vi "Main.vi"() -> ()   [LabVIEW 2014]
doc: "Use this template to build a simple state machine design pattern. Each state executes code and determines which state to transition to."
uses:
  Tipos de onda.ctl
  controls/State.ctl
  controls/Data.ctl
  <vilib>/Waveform/WDTFileIO.llb/ Write Waveform to File.vi
  <vilib>/Analysis/1siggen.llb/Ramp Pattern by Delta.vi
  <vilib>/Waveform/WDTOps.llb/WDT Append Waveforms DBL.vi
  <vilib>/measure/NI_MABase.lvlib
  <vilib>/Waveform/WDTFileIO.llb/Read Waveform from File.vi
  <vilib>/Waveform/WDTFileIO.llb/Export Waveforms To Spreadsheet File (1D).vi
  <vilib>/Analysis/NI_AALBase.lvlib
panel:
  in  "Número de ciclos":dbl
  in  "Tempo de descida":dbl
  in  "Tempo de estabilização":dbl
  in  "Tempo de subida":dbl
  in  "Cortar onda":bool
  in  "Taxa de amostragem":i32
  in  "Amplitude":dbl
  in  "Offset":dbl(slide) scale=0.0..10.0
  out "Ajuste de parâmetros":waveform(dbl)(graph)={"t0"=timestamp(524673.0 s since 1904-01-01), "dt"=0.001, "Y"=[]}
  out "Onda customizada final":waveform(dbl)(graph)
  in  "Duty Cycle (%)":dbl(knob) scale=0.0..100.0
  in  "Fase da onda":dbl(slide) scale=0.0..180.0
  in  "Multiplicador de Frequência":dbl(slide) scale=0.0..1000.0
  in  "Frequência (Hz)":dbl(knob) scale=0.0..10.0
  in  "Tipo de onda":T1
  in  "Gerar nova onda":bool
  in  "Salvar onda":bool
  in  "Histórico de ondas":bool
  in  "Concatenar na onda final":bool
  in  "Sair":bool
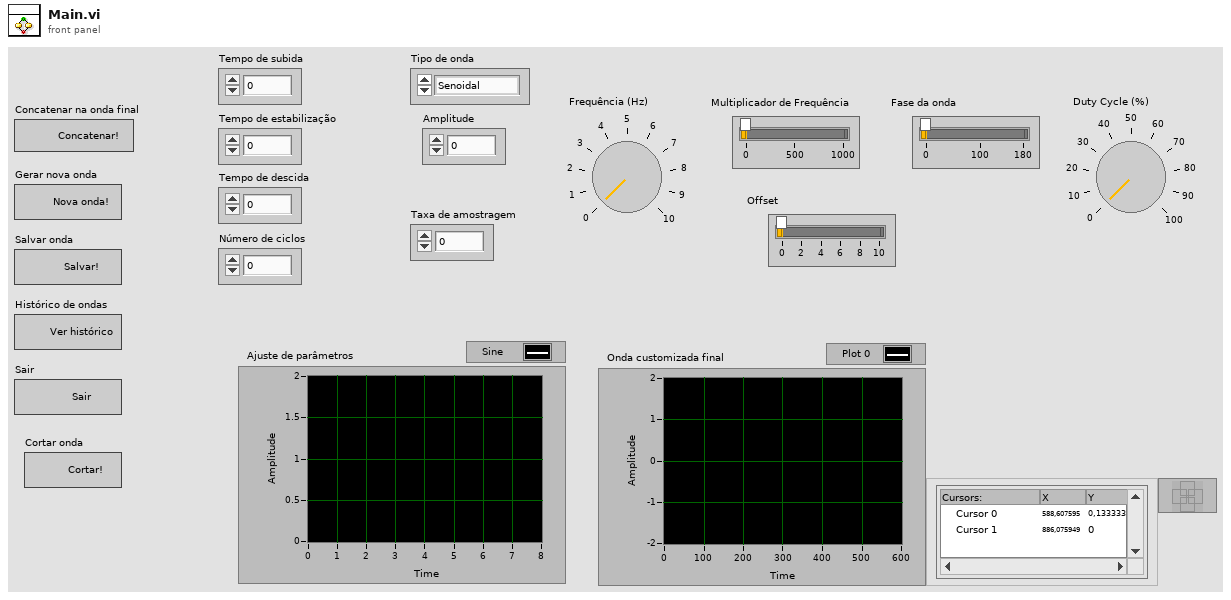
[diagram p1: front panel]
types:
  T1 = typedef "Tipos de onda.ctl" = enum16{"Senoidal", "Quadrada", "Triangular", "Trapezoidal", "Dente de Serra"}
  T2 = typedef "Data.ctl" = cluster{"Boolean <Replace Me>":bool, "String <Replace Me>":string, "Numeric <Replace Me>":dbl, "Onda final":waveform(dbl), "Onda prévia":waveform(dbl), "Tipo de onda":T1, "Frequência (Hz) ":dbl, "Multiplicador de Frequência":dbl, "Fase da onda":dbl, "Duty Cycle (%)":dbl, "Offset":dbl, "Amplitude":dbl, "Taxa de amostragem":i32, "Remove Button":bool, "Tempo de subida":dbl, "Tempo de estabilização":dbl, "Tempo de descida":dbl, "Número de ciclos":dbl}
  T3 = typedef "State.ctl" = enum16{"Inicializar", "Aguardar evento", "Concatenar na onda final", "Ajustar onda prévia", "Cortar onda", "Gerar nova onda", "Salvar onda", "Histórico de ondas", "Sair"}
  T4 = typedef "LVCursorListTypeDef.ctl" = cluster{"Name":string, "Color":u32, "Style":u8, "Point Style":u8, "Name Visible":bool, "Allow Drag":bool, "Cursor Mode":u32, "Plot":i32, "Index":i32, "Position":cluster{"X":dbl, "Y":dbl}, "X Scale":u32, "Y Scale":u32, "Watch Plots":i32[], "Watch All Plots":bool, "Plot Area":i32, "Label Offset":cluster{"X":dbl, "Y":dbl}}[]
  T5 = cluster{"CrsrList[0]":cluster{"Name":string, "Color":u32, "Style":u8, "Point Style":u8, "Name Visible":bool, "Allow Drag":bool, "Cursor Mode":u32, "Plot":i32, "Index":i32, "Position":cluster{"X":dbl, "Y":dbl}, "X Scale":u32, "Y Scale":u32, "Watch Plots":i32[], "Watch All Plots":bool, "Plot Area":i32, "Label Offset":cluster{"X":dbl, "Y":dbl}}, "CrsrList[1]":cluster{"Name":string, "Color":u32, "Style":u8, "Point Style":u8, "Name Visible":bool, "Allow Drag":bool, "Cursor Mode":u32, "Plot":i32, "Index":i32, "Position":cluster{"X":dbl, "Y":dbl}, "X Scale":u32, "Y Scale":u32, "Watch Plots":i32[], "Watch All Plots":bool, "Plot Area":i32, "Label Offset":cluster{"X":dbl, "Y":dbl}}, "CrsrList[2]":cluster{"Name":string, "Color":u32, "Style":u8, "Point Style":u8, "Name Visible":bool, "Allow Drag":bool, "Cursor Mode":u32, "Plot":i32, "Index":i32, "Position":cluster{"X":dbl, "Y":dbl}, "X Scale":u32, "Y Scale":u32, "Watch Plots":i32[], "Watch All Plots":bool, "Plot Area":i32, "Label Offset":cluster{"X":dbl, "Y":dbl}}, "CrsrList[3]":cluster{"Name":string, "Color":u32, "Style":u8, "Point Style":u8, "Name Visible":bool, "Allow Drag":bool, "Cursor Mode":u32, "Plot":i32, "Index":i32, "Position":cluster{"X":dbl, "Y":dbl}, "X Scale":u32, "Y Scale":u32, "Watch Plots":i32[], "Watch All Plots":bool, "Plot Area":i32, "Label Offset":cluster{"X":dbl, "Y":dbl}}, "CrsrList[4]":cluster{"Name":string, "Color":u32, "Style":u8, "Point Style":u8, "Name Visible":bool, "Allow Drag":bool, "Cursor Mode":u32, "Plot":i32, "Index":i32, "Position":cluster{"X":dbl, "Y":dbl}, "X Scale":u32, "Y Scale":u32, "Watch Plots":i32[], "Watch All Plots":bool, "Plot Area":i32, "Label Offset":cluster{"X":dbl, "Y":dbl}}, "CrsrList[5]":cluster{"Name":string, "Color":u32, "Style":u8, "Point Style":u8, "Name Visible":bool, "Allow Drag":bool, "Cursor Mode":u32, "Plot":i32, "Index":i32, "Position":cluster{"X":dbl, "Y":dbl}, "X Scale":u32, "Y Scale":u32, "Watch Plots":i32[], "Watch All Plots":bool, "Plot Area":i32, "Label Offset":cluster{"X":dbl, "Y":dbl}}, "CrsrList[6]":cluster{"Name":string, "Color":u32, "Style":u8, "Point Style":u8, "Name Visible":bool, "Allow Drag":bool, "Cursor Mode":u32, "Plot":i32, "Index":i32, "Position":cluster{"X":dbl, "Y":dbl}, "X Scale":u32, "Y Scale":u32, "Watch Plots":i32[], "Watch All Plots":bool, "Plot Area":i32, "Label Offset":cluster{"X":dbl, "Y":dbl}}, "CrsrList[7]":cluster{"Name":string, "Color":u32, "Style":u8, "Point Style":u8, "Name Visible":bool, "Allow Drag":bool, "Cursor Mode":u32, "Plot":i32, "Index":i32, "Position":cluster{"X":dbl, "Y":dbl}, "X Scale":u32, "Y Scale":u32, "Watch Plots":i32[], "Watch All Plots":bool, "Plot Area":i32, "Label Offset":cluster{"X":dbl, "Y":dbl}}, "CrsrList[8]":cluster{"Name":string, "Color":u32, "Style":u8, "Point Style":u8, "Name Visible":bool, "Allow Drag":bool, "Cursor Mode":u32, "Plot":i32, "Index":i32, "Position":cluster{"X":dbl, "Y":dbl}, "X Scale":u32, "Y Scale":u32, "Watch Plots":i32[], "Watch All Plots":bool, "Plot Area":i32, "Label Offset":cluster{"X":dbl, "Y":dbl}}}
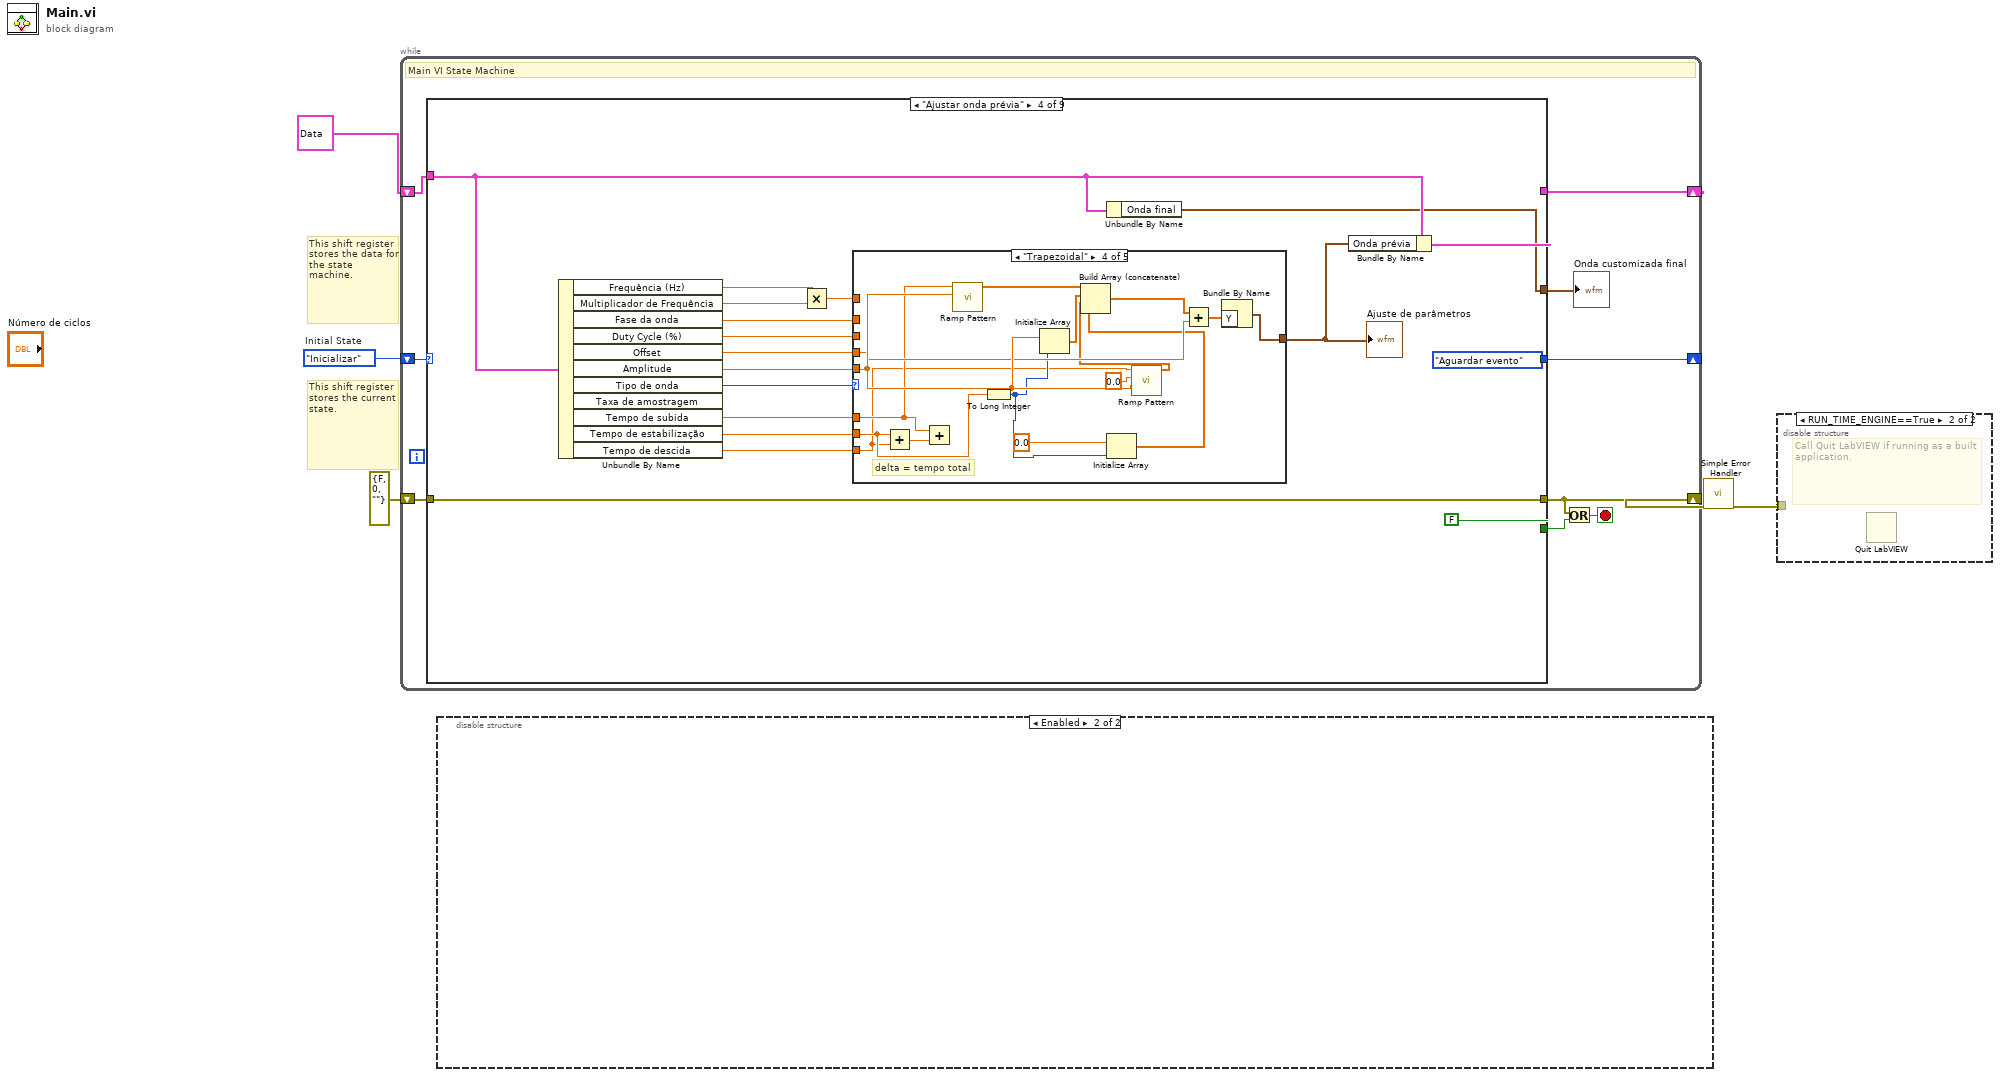
[diagram p0: block diagram]
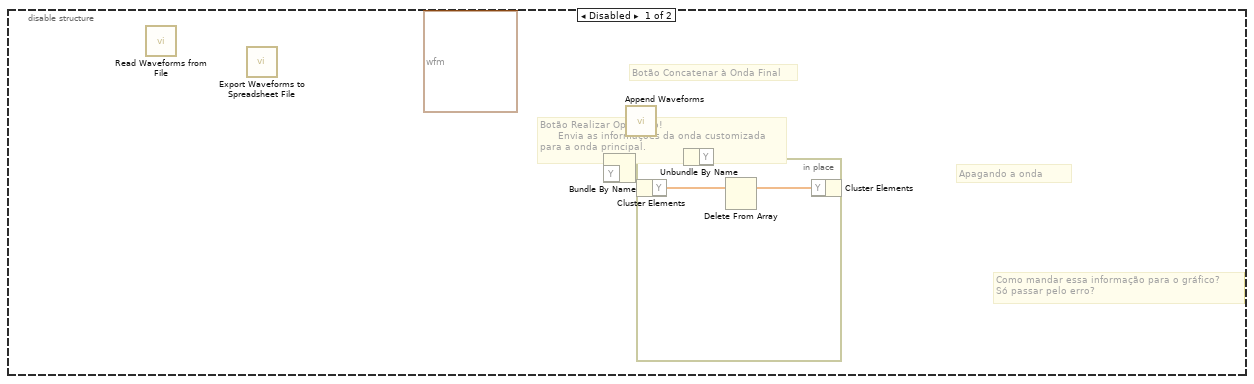
[diagram p2: hidden frame]
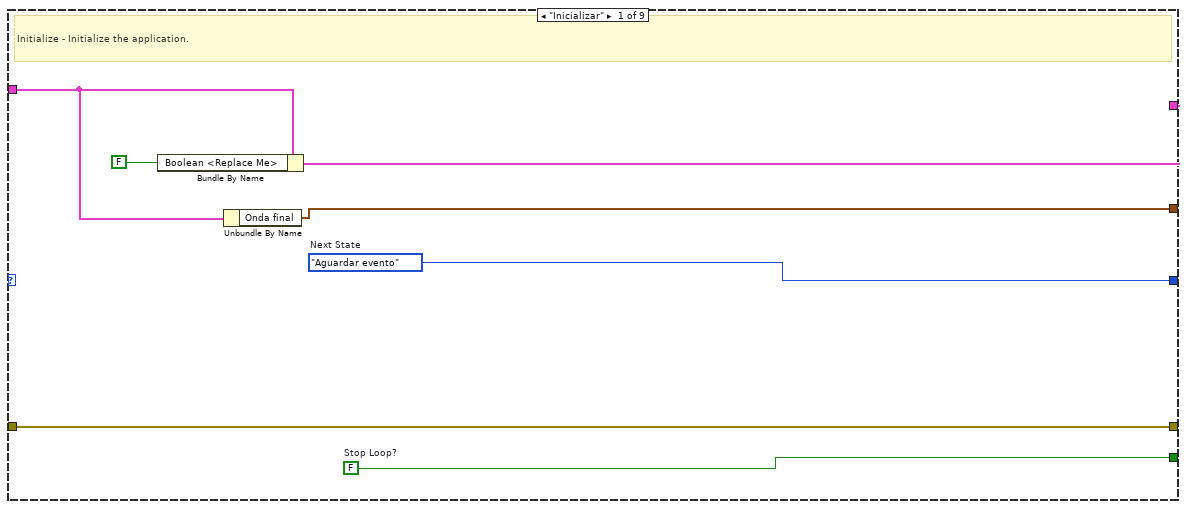
[diagram p4: hidden frame]
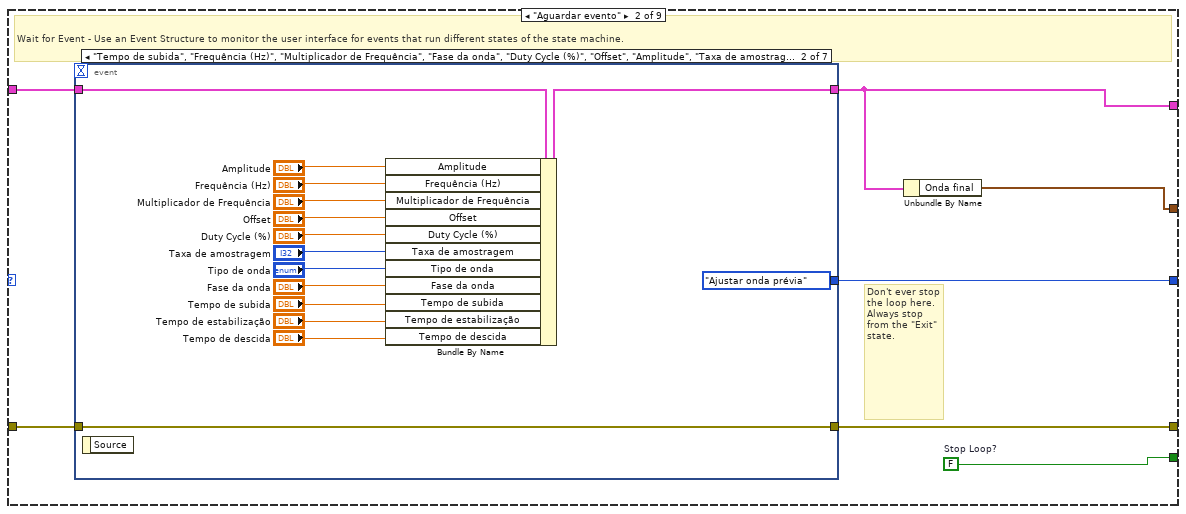
[diagram p5: hidden frame]
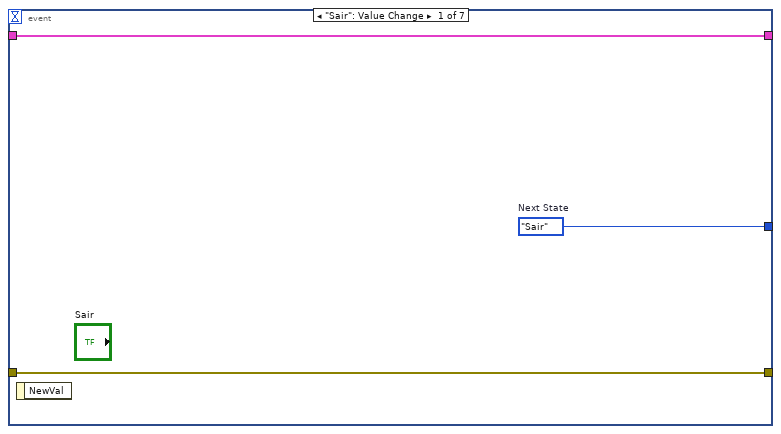
[diagram p6: hidden frame]
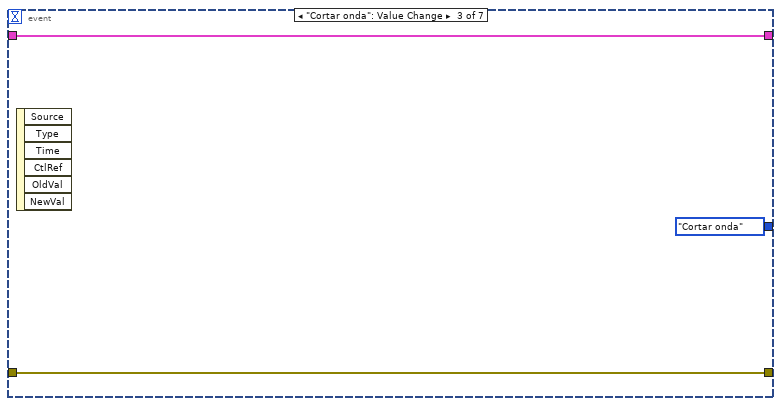
[diagram p7: hidden frame]
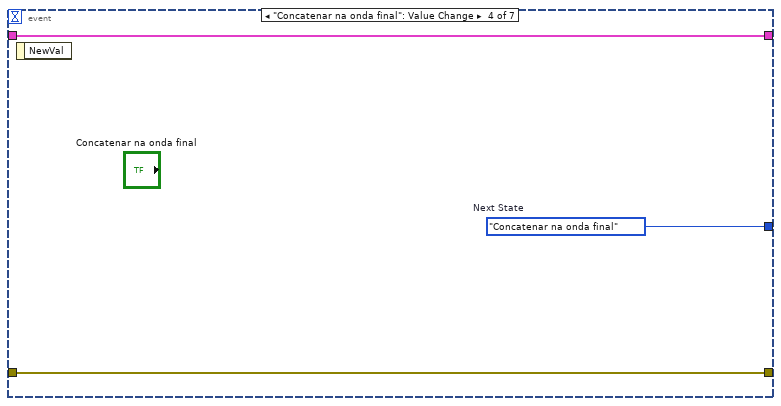
[diagram p8: hidden frame]
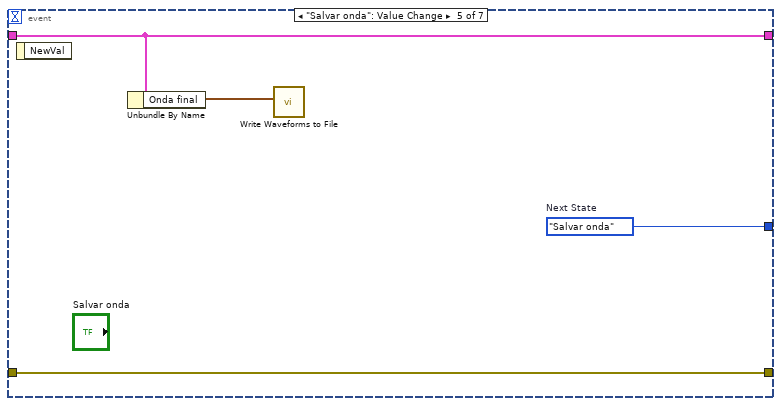
[diagram p9: hidden frame]
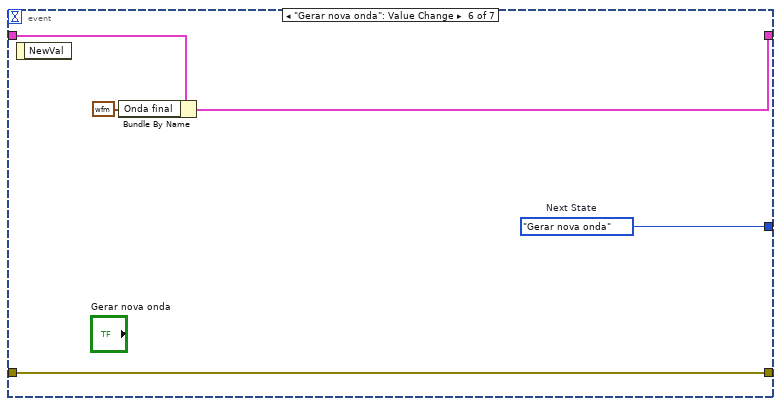
[diagram p10: hidden frame]
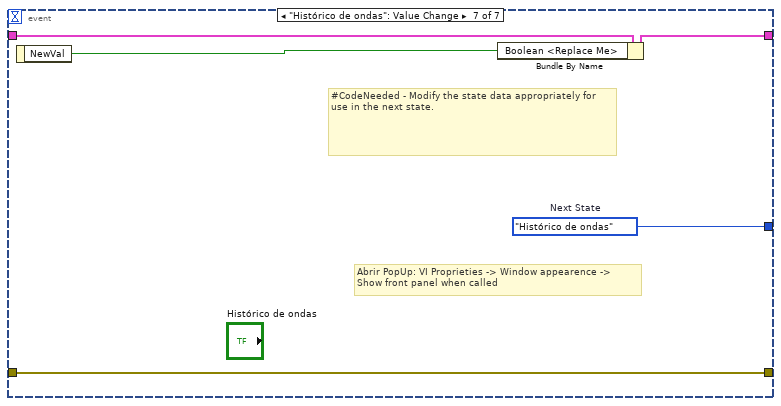
[diagram p11: hidden frame]
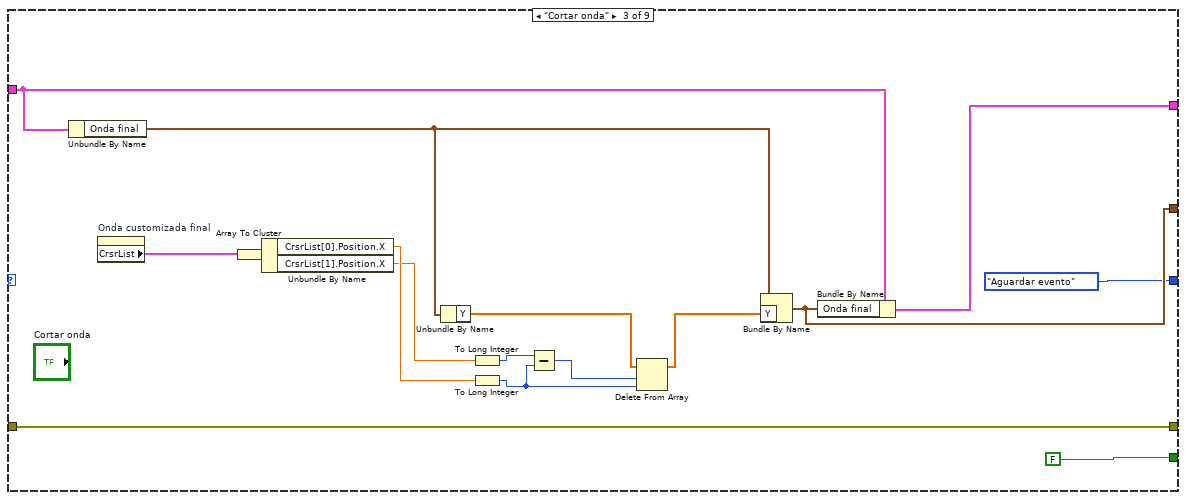
[diagram p12: hidden frame]
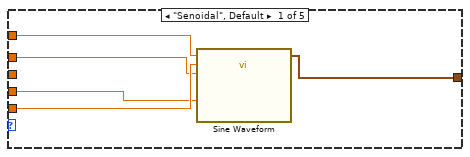
[diagram p13: hidden frame]
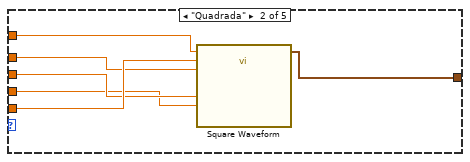
[diagram p14: hidden frame]
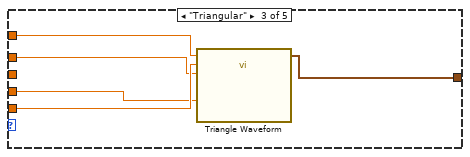
[diagram p15: hidden frame]
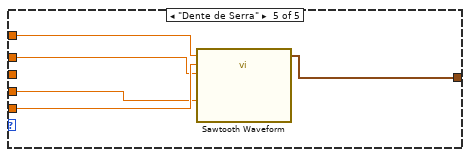
[diagram p16: hidden frame]
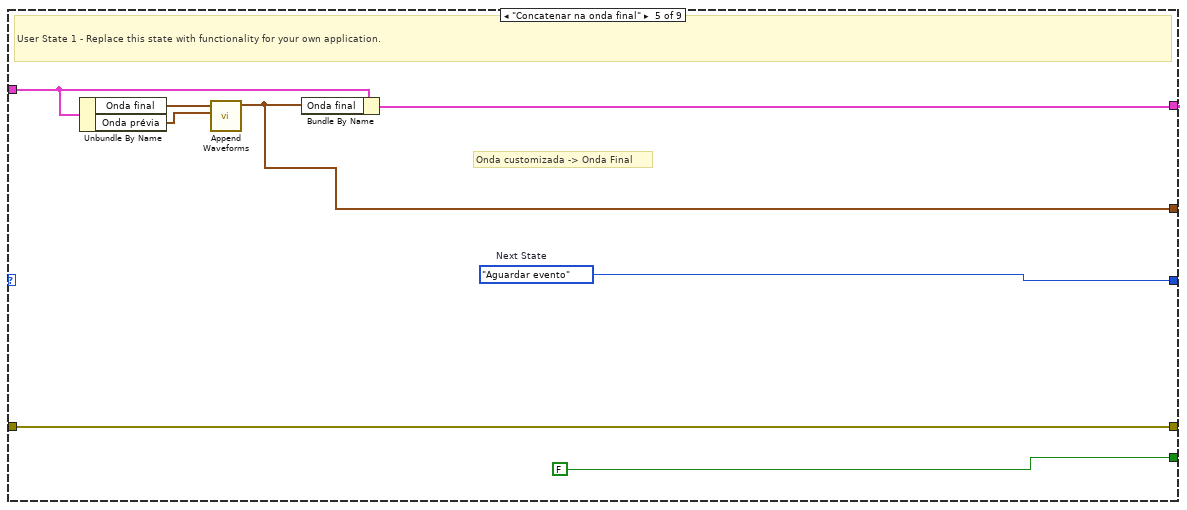
[diagram p17: hidden frame]
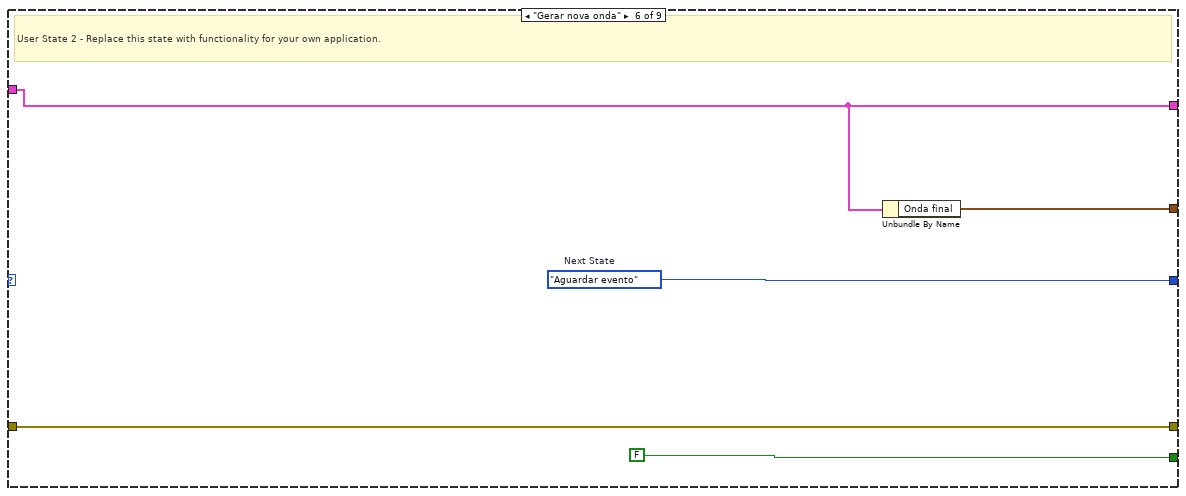
[diagram p18: hidden frame]
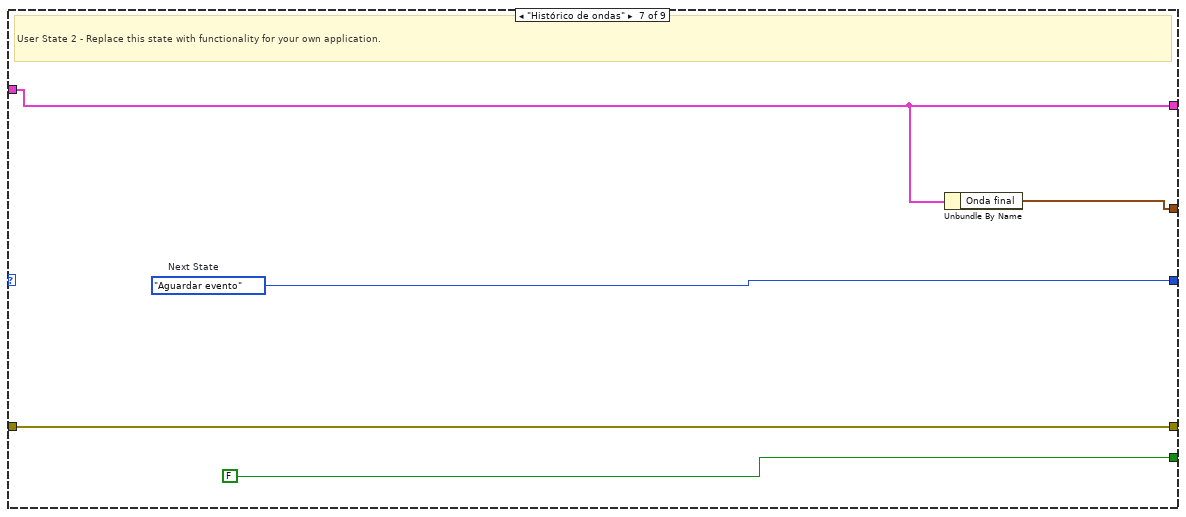
[diagram p19: hidden frame]
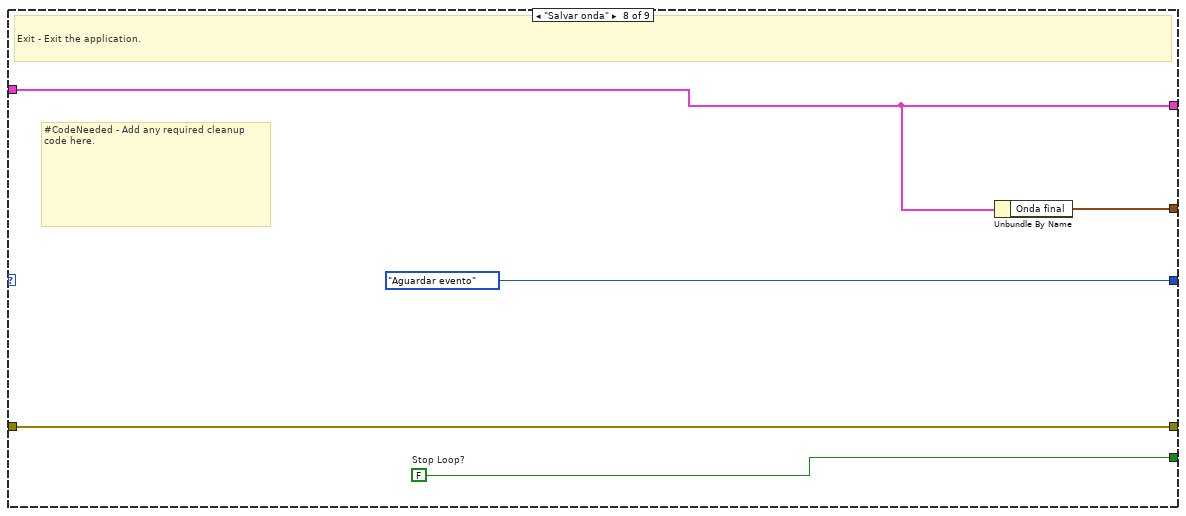
[diagram p20: hidden frame]
diagram:
  w5 = State."Inicializar"  # Initial State
  # "This shift register stores the data for the state machine."
  # "This shift register stores the current state."
  n1 = while {
    shift-right: [w13] -> _
    shift-left: w5 -> [w14]
    shift-right: [w11] -> _
    shift-left: T2 {"Boolean <Replace Me>"=FALSE, "String <Replace Me>"="", "Numeric <Replace Me>"=0.0, "Onda final"={"t0"=timestamp(0 s since 1904-01-01), "dt"=1.0, "Y"=[]}, "Onda prévia"={"t0"=timestamp(0 s since 1904-01-01), "dt"=1.0, "Y"=[]}, "Tipo de onda"=enum."Senoidal", "Frequência (Hz) "=0.0, "Multiplicador de Frequência"=0.0, "Fase da onda"=0.0, "Duty Cycle (%)"=0.0, "Offset"=0.0, "Amplitude"=0.0, "Taxa de amostragem"=0, "Remove Button"=FALSE, "Tempo de subida"=0.0, "Tempo de estabilização"=0.0, "Tempo de descida"=0.0, "Número de ciclos"=0.0} ("Data") -> [w12]
    shift-right: [w8] -> w2
    shift-left: errorcluster {"status"=FALSE, "code"=0, "source"=""} ("error constant") -> [w10]
    stop <- w9 stop-if-true
    # "Main VI State Machine"
    n2 = case shown="\"Ajustar onda prévia\"" w14 {
      tunnel: [w21 w28 State."Aguardar evento" ("(Value Not Used)") State."Aguardar evento" ("(Value Not Used)") w145 w150 w155 State."Aguardar evento" w165] -> w13
      tunnel: [w20 w27 FALSE ("Stop Loop?") FALSE FALSE ("Stop Loop?") FALSE ("Stop Loop?") FALSE ("Stop Loop?") w159 w164] -> w7
      tunnel: w12 -> [w16 w26 w71 w90 w139 w146 w151 w156 w161]
      tunnel: [w19 w23 w70 w94 w142 w146 w151 w156 w161] -> w11
      tunnel: w10 -> [w17 w24 w79 w100 w143 w148 w153 w158 w163]
      tunnel: [w17 w25 w79 w100 w143 w148 w153 w158 w163] -> w8
      tunnel: [w15 w22 w69 w89 w138 w147 w152 w157 w162] -> w6
      frame "Inicializar" {
        w20 = FALSE  # Stop Loop?
        w21 = State."Aguardar evento"  # Next State
        # "Initialize - Initialize the application."
        n3 = Bundle By Name(cluster=w16, "Boolean <Replace Me>"=FALSE ("Replace_Me_Boolean")) -> (w19:T2)
        n4 = Unbundle By Name(w16) -> ("Onda final"=w15:waveform(dbl))
      }
      frame "Aguardar evento" {
        w27 = FALSE  # Stop Loop?
        # "Don't ever stop the loop here. Always stop from the \"Exit\" state."
        # "Wait for Event - Use an Event Structure to monitor the user interface for events that run different states of the state machine."
        n5 = event shown="[1] \"Tempo de subida\", \"Frequência (Hz)\", \"Multiplicador de Frequência\", \"Fase da onda\", \"Duty Cycle (%)\", \"Offset\", \"Amplitude\", \"Taxa de amostragem\", \"Tempo de estabilização\", \"Tempo de descida\": Value Change" {
          selector: _ -> [_ _ _ _ _ _ _]
          dyn-events: _ -> [_ _ _ _ _ _ _]
          timeout: _ -> [_ _ _ _ _ _ _]
          tunnel: [w31 State."Ajustar onda prévia" ("Next State") State."Cortar onda" ("Next State") w52 w56 w61 w66] -> w28
          tunnel: w26 -> [w30 w46 w49 w50 w53 w59 w65]
          tunnel: [w30 w43 w49 w50 w53 w57 w64] -> w23
          tunnel: w24 -> [w29 w45 w48 w51 w55 w60 w63]
          tunnel: [w29 w45 w48 w51 w55 w60 w63] -> w25
          event "Sair": Value Change {
            w31 = State."Sair"  # Next State
            n6 = event-data() -> ()  [unwired: 1 in, 1 out]
          }
          event "Tempo de subida", "Frequência (Hz)", "Multiplicador de Frequência", "Fase da onda", "Duty Cycle (%)", "Offset", "Amplitude", "Taxa de amostragem", "Tempo de estabilização", "Tempo de descida": Value Change {
            n7 = event-data() -> ()  [unwired: 1 in, 1 out]
            n8 = Bundle By Name(cluster=w46, "Amplitude"="Amplitude", "Frequência (Hz)"="Frequência (Hz)", "Multiplicador de Frequência"="Multiplicador de Frequência", "Offset"="Offset", "Duty Cycle (%)"="Duty Cycle (%)", "Taxa de amostragem"="Taxa de amostragem", "Tipo de onda"="Tipo de onda", "Fase da onda"="Fase da onda", "Tempo de subida"="Tempo de subida", "Tempo de estabilização"="Tempo de estabilização", "Tempo de descida"="Tempo de descida") -> (w43:T2)
          }
          event "Cortar onda": Value Change {
            n9 = event-data() -> ()  [unwired: 1 in, 6 out]
          }
          event "Concatenar na onda final": Value Change {
            w52 = State."Concatenar na onda final"  # Next State
            n10 = event-data() -> ()  [unwired: 1 in, 1 out]
          }
          event "Salvar onda": Value Change {
            w56 = State."Salvar onda"  # Next State
            n11 = event-data() -> ()  [unwired: 1 in, 1 out]
            n12 = Unbundle By Name(w53) -> ("Onda final"=w54:waveform(dbl))
            n13 = call-poly <vilib>:"Write Waveforms to File.vi"("waveform"=w54) -> ()  [unwired: 9 in, 2 out]
          }
          event "Gerar nova onda": Value Change {
            w61 = State."Gerar nova onda"  # Next State
            n14 = event-data() -> ()  [unwired: 1 in, 1 out]
            n15 = Bundle By Name(cluster=w59, "Onda final"=waveform(dbl) {"t0"=timestamp(0 s since 1904-01-01), "dt"=1.0, "Y"=[]}) -> (w57:T2)
          }
          event "Histórico de ondas": Value Change {
            w66 = State."Histórico de ondas"  # Next State
            # "Abrir PopUp: VI Proprieties -> Window appearence ->\nShow front panel when called"
            # "#CodeNeeded - Modify the state data appropriately for use in the next state."
            n16 = event-data() -> ("NewVal"=w62:bool)  [unwired: 1 in]
            n17 = Bundle By Name(cluster=w65, "Boolean <Replace Me>"=w62) -> (w64:T2)
          }
        }
        n18 = Unbundle By Name(w23) -> ("Onda final"=w22:waveform(dbl))
      }
      frame "Cortar onda" {
        n19 = Unbundle By Name(w71) -> ("Onda final"=w72:waveform(dbl))
        n20 = property on="Onda customizada final" class="WFGraph (strict)"() -> ("CrsrList"=w81:T4)  [unwired: 2 in, 2 out]
        n21 = Array To Cluster(array=w81) -> (cluster=w80:T5)
        n22 = Unbundle By Name(w80) -> ("CrsrList[0].Position.X"=w78:dbl, "CrsrList[1].Position.X"=w77:dbl)
        n23 = Unbundle By Name(w72) -> ("Y"=w82:dbl[])
        n24 = To Long Integer(number=w77) -> (32bit integer=w76:i32)
        n25 = To Long Integer(number=w78) -> (32bit integer=w75:i32)
        n26 = Subtract(x=w76, y=w75) -> (x-y=w74:i32)
        n27 = Delete From Array(array=w82, length=w74, index=w75) -> (array with subset deleted=w73:dbl[])  [unwired: 1 out]
        n28 = Bundle By Name(cluster=w72, "Y"=w73) -> (w69:waveform(dbl))
        n29 = Bundle By Name(cluster=w71, "Onda final"=w69) -> (w70:T2)
      }
      frame "Ajustar onda prévia" {
        n30 = Unbundle By Name(w90) -> ("Frequência (Hz)"=w88:dbl, "Multiplicador de Frequência"=w87:dbl, "Fase da onda"=w93:dbl, "Duty Cycle (%)"=w92:dbl, "Offset"=w91:dbl, "Amplitude"=w98:dbl, "Tipo de onda"=w99:T1, "Tempo de subida"=w85:dbl, "Tempo de estabilização"=w84:dbl, "Tempo de descida"=w83:dbl)  [unwired: 1 out]
        n31 = Multiply(x=w88, y=w87) -> (x*y=w86:dbl)
        n32 = case shown="\"Trapezoidal\"" w99 {
          tunnel: [w105 w111 w116 w127 w137] -> w95
          tunnel: w98 -> [w104 w110 w115 w130 w136]
          tunnel: w86 -> [w103 w109 w114 _ w135]
          tunnel: w93 -> [w102 w108 w113 _ w134]
          tunnel: w92 -> [_ w107 _ _ _]
          tunnel: w91 -> [w101 w106 w112 w128 w133]
          tunnel: w85 -> [_ _ _ w118 _]
          tunnel: w84 -> [_ _ _ w131 _]
          tunnel: w83 -> [_ _ _ w117 _]
          frame "Senoidal", Default {
            n33 = call <vilib>:"Sine Waveform.vi"("offset"=w101, "phase"=w102, "amplitude"=w104, "frequency"=w103) -> ("signal out"=w105:waveform(dbl))  [unwired: 6 in, 1 out]
          }
          frame "Quadrada" {
            n34 = call <vilib>:"Square Waveform.vi"("duty cycle (%)"=w107, "offset"=w106, "phase"=w108, "amplitude"=w110, "frequency"=w109) -> ("signal out"=w111:waveform(dbl))  [unwired: 5 in, 1 out]
          }
          frame "Triangular" {
            n35 = call <vilib>:"Triangle Waveform.vi"("offset"=w112, "phase"=w113, "amplitude"=w115, "frequency"=w114) -> ("signal out"=w116:waveform(dbl))  [unwired: 6 in, 1 out]
          }
          frame "Trapezoidal" {
            # "delta = tempo total"
            n36 = Add(x=w131, y=w117) -> (x+y=w132:dbl)
            n37 = Add(x=w118, y=w132) -> ()  [unwired: 1 out]
            n38 = call-poly <vilib>:"Ramp Pattern.vi"("end"=w130, "delta"=w118) -> ("Ramp Pattern"=w126:dbl[])  [unwired: 7 in, 2 out]
            n39 = To Long Integer(number=w131) -> (32bit integer=w120:i32)
            n40 = Initialize Array(w130, w120) -> (w125:dbl[])
            n41 = Initialize Array(0.0 ("element"), w120) -> (w119:dbl[])
            n42 = call-poly <vilib>:"Ramp Pattern.vi"("start"=w130, "end"=0.0, "delta"=w117) -> ("Ramp Pattern"=w124:dbl[])  [unwired: 6 in, 2 out]
            n43 = Build Array (concatenate)(w126, w125, w124, w119) -> (w123:dbl[])
            n44 = Add(x=w123, y=w128) -> (x+y=w122:dbl[])
            n45 = Bundle By Name("Y"=w122) -> (w127:waveform(dbl))  [unwired: 1 in]
          }
          frame "Dente de Serra" {
            n46 = call <vilib>:"Sawtooth Waveform.vi"("offset"=w133, "phase"=w134, "amplitude"=w136, "frequency"=w135) -> ("signal out"=w137:waveform(dbl))  [unwired: 6 in, 1 out]
          }
        }
        "Ajuste de parâmetros" <- w95
        n47 = Unbundle By Name(w90) -> ("Onda final"=w89:waveform(dbl))
        n48 = Bundle By Name(cluster=w90, "Onda prévia"=w95) -> (w94:T2)
      }
      frame "Concatenar na onda final" {
        w145 = State."Aguardar evento"  # Next State
        # "Onda customizada -> Onda Final"
        # "User State 1 - Replace this state with functionality for your own application."
        n49 = Unbundle By Name(w139) -> ("Onda final"=w141:waveform(dbl), "Onda prévia"=w140:waveform(dbl))
        n50 = call-poly <vilib>:"Append Waveforms.vi"("waveform B"=w140, "waveform A"=w141) -> ("waveform out"=w138:waveform(dbl))  [unwired: 8 in, 1 out]
        n51 = Bundle By Name(cluster=w139, "Onda final"=w138) -> (w142:T2)
      }
      frame "Gerar nova onda" {
        w150 = State."Aguardar evento"  # Next State
        # "User State 2 - Replace this state with functionality for your own application."
        n52 = Unbundle By Name(w146) -> ("Onda final"=w147:waveform(dbl))
      }
      frame "Histórico de ondas" {
        w155 = State."Aguardar evento"  # Next State
        # "User State 2 - Replace this state with functionality for your own application."
        n53 = Unbundle By Name(w151) -> ("Onda final"=w152:waveform(dbl))
      }
      frame "Salvar onda" {
        w159 = FALSE  # Stop Loop?
        # "#CodeNeeded - Add any required cleanup code here."
        # "Exit - Exit the application."
        n54 = Unbundle By Name(w156) -> ("Onda final"=w157:waveform(dbl))
      }
      frame "Sair" {
        w164 = TRUE  # Stop Loop?
        w165 = State."Sair"  # (Value Not Used)
        # "Exit - Exit the application."
        n55 = Unbundle By Name(w161) -> ("Onda final"=w162:waveform(dbl))
      }
    }
    "Onda customizada final" <- w6
    n56 = Or(x=w8, y=w7) -> (x .or. y?=w9:bool)
  }
  n57 = disable-structure shown="Enabled" {
    frame Disabled {
      (unwired) waveform(dbl) {"t0"=timestamp(0 s since 1904-01-01), "dt"=1.0, "Y"=[]} ("Waveform")
      # "Botão Concatenar à Onda Final"
      # "Como mandar essa informação para o gráfico?\nSó passar pelo erro?"
      # "Apagando a onda"
      # "Botão Realizar Operação!\n      Envia as informações da onda customizada\npara a onda principal."
      n58 = call-poly <vilib>:"Read Waveforms from File.vi"() -> ()  [unwired: 6 in, 4 out]
      n59 = call-poly <vilib>:"Export Waveforms to Spreadsheet File.vi"() -> ()  [unwired: 10 in, 2 out]
      n60 = Bundle By Name() -> ()  [unwired: 2 in, 1 out]
      n61 = call-poly <vilib>:"Append Waveforms.vi"() -> ()  [unwired: 10 in, 2 out]
      n62 = in-place {
        n63 = in-place-cluster #1() -> ("Y"=w167:dbl[])  [unwired: 1 in]
        n64 = Delete From Array(array=w167) -> (array with subset deleted=w166:dbl[])  [unwired: 2 in, 1 out]
        n65 = in-place-cluster #1("Y"=w166) -> ()  [unwired: 1 out]
      }
      n66 = Unbundle By Name() -> ()  [unwired: 1 in, 1 out]
    }
    frame Enabled {
    }
  }
  n67 = call <vilib>:"Simple Error Handler.vi"("error in (no error)"=w2) -> ("error out"=w1:errorcluster)  [unwired: 4 in, 4 out]
  n68 = disable-structure shown="RUN_TIME_ENGINE==True" {
    disable-tunnel: w1 -> [_ _]
    frame condition #0 (active) {
    }
    frame condition #1 {
      # "Call Quit LabVIEW if running as a built application."
      n69 = Quit LabVIEW() -> ()  [unwired: 1 in]
    }
  }
